vi "Acquire image (SubVI).vi"(9 "Buffer number":i32, 10 "Camera type":T4(ring), 11 "Measurement camera \ncluster in":T3) -> (1 "Image Out":T1, 2 "Measurement camera cluster out":T3, 4 "Buffer Number Out":u32)   [LabVIEW 2012]
uses:
  <vilib>/userdefined/High Color/IMAQdx.ctl
  <vilib>/vision/Image Controls.llb/IMAQ Image.ctl
  <vilib>/vision/driver/NI_Vision_Acquisition_Software.lvlib
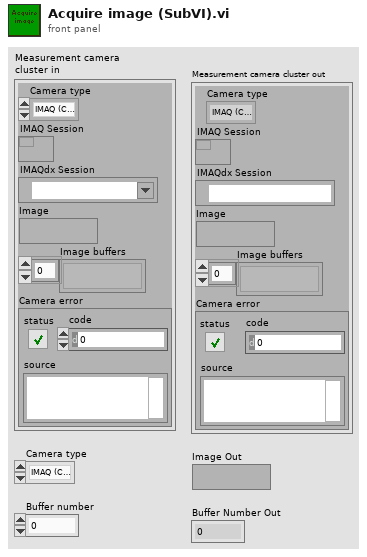
[diagram p1: front panel]
types:
  T1 = typedef "IMAQ Image.ctl" = refnum<image>
  T2 = typedef "IMAQdx.ctl" = refnum<k21>
  T3 = cluster{"Camera type":enum16{"IMAQ (Camera Link)", "IMAQ ring", "IMAQdx (firewire)", "No camera"}, "IMAQ Session":refnum<k11>, "IMAQdx Session":T2, "Image":T1, "Image buffers":T1[], "Camera error":errorcluster}
  T4 = enum16{"IMAQ (Camera Link)", "IMAQ ring", "IMAQdx (firewire)", "No camera"}
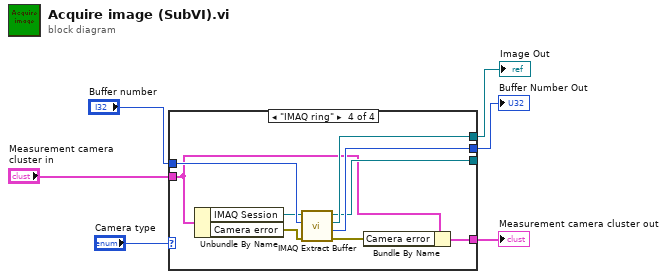
[diagram p0: block diagram]
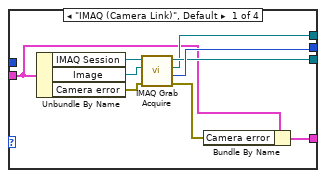
[diagram p2: hidden frame]
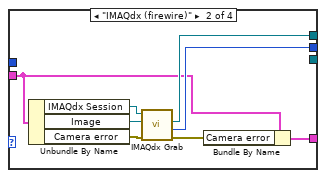
[diagram p3: hidden frame]
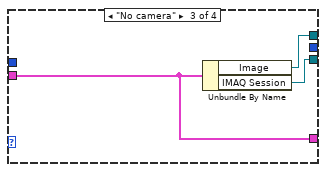
[diagram p4: hidden frame]
diagram:
  n1 = case shown="\"IMAQ ring\"" "Camera type" {
    tunnel: "Measurement camera \ncluster in" -> [w10 w18 w24 w29]
    tunnel: [w15 w23 _ w33] -> w1
    tunnel: "Buffer number" -> [_ _ _ w34]
    tunnel: [w11 w19 w26 w32] -> w3
    tunnel: [w12 _ w25 w30] -> _
    tunnel: [w9 w17 w24 w27] -> w5
    frame "IMAQ (Camera Link)", Default {
      n2 = Unbundle By Name(w10) -> ("IMAQ Session"=w7:refnum<k11>, "Image"=w14:T1, "Camera error"=w13:errorcluster)
      n3 = call <vilib>:"IMAQ Grab Acquire.vi"("error in (no error)"=w13, "Image In"=w14, "IMAQ Session In"=w7) -> ("error out"=w8:errorcluster, "Acquired Buffer Number"=w15:u32, "Image Out"=w11:T1, "IMAQ Session Out"=w12:refnum<k11>)  [unwired: 5 in]
      n4 = Bundle By Name(cluster=w10, "Camera error"=w8) -> (w9:T3)
    }
    frame "IMAQdx (firewire)" {
      n5 = Unbundle By Name(w18) -> ("IMAQdx Session"=w22:T2, "Image"=w21:T1, "Camera error"=w20:errorcluster)
      n6 = call <vilib>:"IMAQdx Grab.vi"("error in"=w20, "Image In"=w21, "Session In"=w22) -> ("error out"=w16:errorcluster, "Buffer Number Out"=w23:u32, "Image Out"=w19:T1)  [unwired: 5 in, 1 out]
      n7 = Bundle By Name(cluster=w18, "Camera error"=w16) -> (w17:T3)
    }
    frame "No camera" {
      n8 = Unbundle By Name(w24) -> ("Image"=w26:T1, "IMAQ Session"=w25:refnum<k11>)
    }
    frame "IMAQ ring" {
      n9 = Unbundle By Name(w29) -> ("IMAQ Session"=w31:refnum<k11>, "Camera error"=w35:errorcluster)
      n10 = call <vilib>:"IMAQ Extract Buffer.vi"("error in (no error)"=w35, "Buffer to extract"=w34, "IMAQ Session In"=w31) -> ("error out"=w28:errorcluster, "Buffer Number"=w33:i32, "Image Out"=w32:T1, "IMAQ Session Out"=w30:refnum<k11>)  [unwired: 3 in, 2 out]
      n11 = Bundle By Name(cluster=w29, "Camera error"=w28) -> (w27:T3)
    }
  }
  "Measurement camera cluster out" <- w5
  "Image Out" <- w3
  "Buffer Number Out" <- w1
